vi "PH_Img_BaseClass.Set GUI Refs.vi"(0 "i ref in":refnum<vi>, 1 "Class":string, 2 "GUI Refs":T1, 5 "error in (no error)":errorcluster) -> (14 "i ref out":refnum<vi>, 19 "error out":errorcluster)   [LabVIEW 2014, in "PH_Img_BaseClass.lvlib"]
uses:
  PH_Img_BaseClass.lvlib
  PH_Img_BaseClass.GUI Refs.ctl
  PH_Common/PH_Common.lvlib
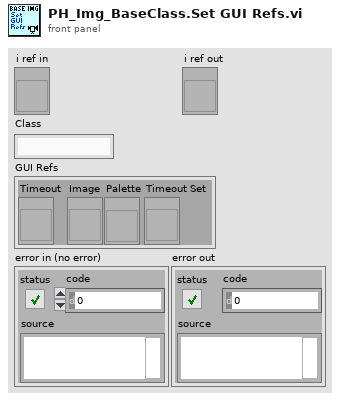
[diagram p1: front panel]
types:
  T1 = typedef "PH_Img_BaseClass.lvlib/PH_Img_BaseClass.GUI Refs.ctl" = cluster{"Timeout":refnum<vi>, "Image":refnum<vi>, "Palette":refnum<vi>, "Timeout Set":refnum<vi>}
  T2 = typedef "PH_Img_BaseClass.lvlib/PH_Img_BaseClass.i attribute.ctl" = cluster{"GUI Refs":T1, "Timeout Image [ms]":i32, "Default Periodic Period [ms]":i32, "Camera":cluster{"Instancename":string, "Notifier":refnum<notifier>}, "Palette":T3, "Cam Settings":cluster{"Cam ID":string, "Gain":dbl, "Brightness":dbl, "Shutter":dbl, "Cam Info Failure":bool, "Mode":i32}}
  T3 = typedef "PH_Img_BaseClass.lvlib/PH_Img_BaseClass.Palette.ctl" = i32
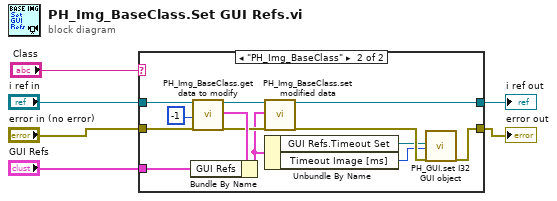
[diagram p0: block diagram]
diagram:
  n1 = case shown="\"PH_Img_BaseClass\"" "Class" {
    tunnel: [w7 w12] -> w6
    tunnel: "error in (no error)" -> [w7 w17]
    tunnel: [w8 w16] -> w4
    tunnel: "i ref in" -> [w8 w14]
    tunnel: "GUI Refs" -> [_ w13]
    frame Default {
    }
    frame "PH_Img_BaseClass" {
      n2 = call "PH_Img_BaseClass.get data to modify.vi"("i ref in"=w14, "ms timeout (10000)"=-1, "error in (no error)"=w17) -> ("i ref out"=w15:refnum<vi>, "i attribute"=w21:T2, "error out"=w18:errorcluster)  [unwired: 13 in, 1 out]
      n3 = Bundle By Name(cluster=w21, "GUI Refs"=w13) -> (w11:T2)
      n4 = call "PH_Img_BaseClass.set modified data.vi"("i ref in"=w15, "i attribute"=w11, "error in (no error)"=w18) -> ("i ref out"=w16:refnum<vi>, "error out"=w19:errorcluster)  [unwired: 15 in]
      n5 = Unbundle By Name(w11) -> ("GUI Refs.Timeout Set"=w10:refnum<vi>, "Timeout Image [ms]"=w9:i32)
      n6 = call "PH_GUI.set I32 GUI object.vi"("I32 GUI Ref"=w10, "value"=w9, "error in (no error)"=w19) -> ("error out"=w12:errorcluster)  [unwired: 16 in]
    }
  }
  "error out" <- w6
  "i ref out" <- w4
